vi "Order Ctlrs and Indis.vi"(8 "Error In":errorcluster, 11 "Connector Pane Object Refs":refnum<vi>[][](array[refnum])) -> (0 "Error Out":errorcluster, 2 "Ordered  Indicators":refnum<vi>[](array[refnum]), 3 "Ordered Controls":refnum<vi>[](array[refnum]))   [LabVIEW 2014]
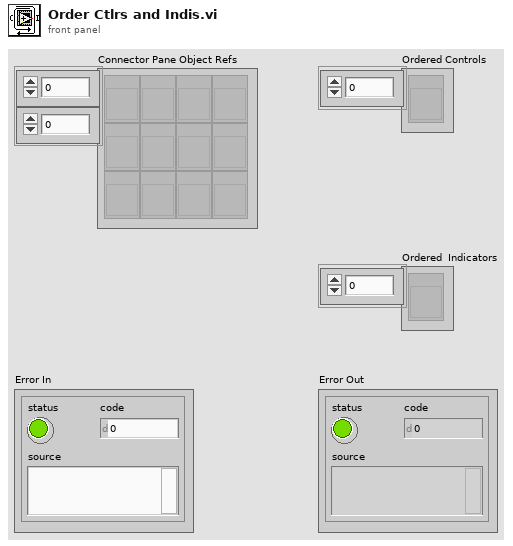
[diagram p1: front panel]
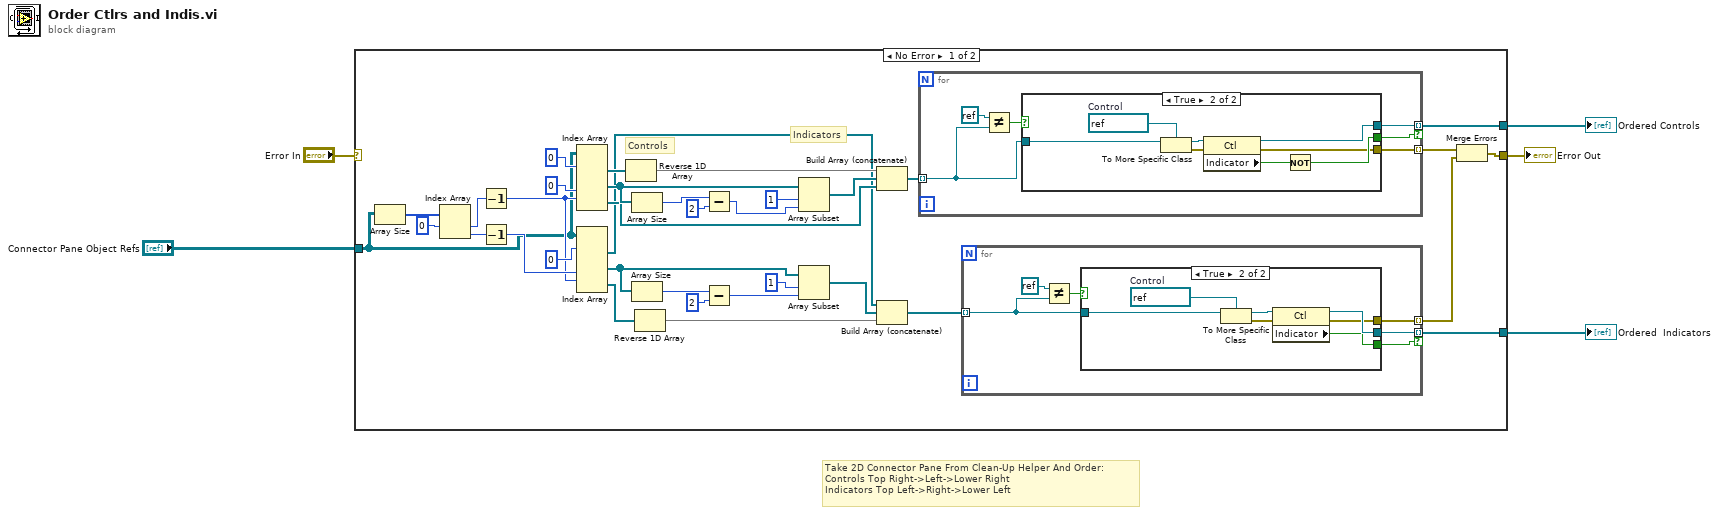
[diagram p0: block diagram]
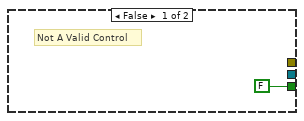
[diagram p2: hidden frame]
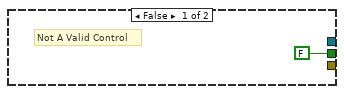
[diagram p3: hidden frame]
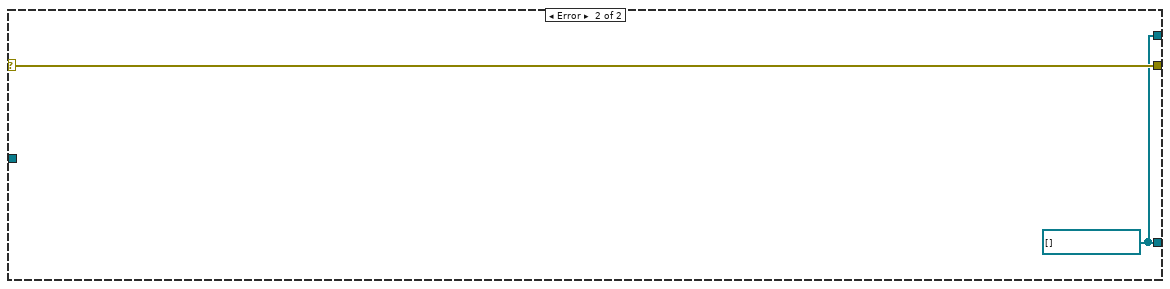
[diagram p4: hidden frame]
diagram:
  # "Take 2D Connector Pane From Clean-Up Helper And Order:\nControls Top Right->Left->Lower Right\nIndicators Top Left->Right->Lower Left"
  n1 = case shown="No Error" "Error In" {
    selector: "Error In" -> [_ w71]
    tunnel: "Connector Pane Object Refs" -> [w13 _]
    tunnel: [w8 w70] -> w4
    tunnel: [w7 w70] -> w3
    tunnel: [w6 w71] -> w1
    frame No Error {
      # "Indicators"
      # "Controls"
      n2 = Array Size(array=w13) -> (size(s)=w32:i32[])
      n3 = Index Array(array=w32, index #1=0 ("index")) -> (element #1=w30:i32, element #2=w25:i32)  [unwired: 1 in]
      n4 = Decrement(x=w30) -> (x-1=w18:i32)
      n5 = Decrement(x=w25) -> (x-1=w24:i32)
      n6 = Index Array(array=w13, index (row) #1=0 ("index (row)"), index (col) #2=0 ("disabled index (col)"), index (row) #3=w18) -> (element #1=w39:refnum<vi>[], element #2=w36:refnum<vi>[], element #3=w27:refnum<vi>[])  [unwired: 3 in]
      n7 = Index Array(array=w13, index (row) #1=0 ("index (row)"), index (col) #2=w24, index (row) #3=w18) -> (element #1=w16:refnum<vi>[], element #2=w19:refnum<vi>[], element #3=w17:refnum<vi>[])  [unwired: 3 in]
      n8 = Reverse 1D Array(array=w39) -> (reversed array=w29:refnum<vi>[])
      n9 = Array Size(array=w36) -> (size(s)=w35:i32)
      n10 = Array Size(array=w19) -> (size(s)=w21:i32)
      n11 = Reverse 1D Array(array=w17) -> (reversed array=w14:refnum<vi>[])
      n12 = Subtract(x=w35, y=2) -> (x-y=w33:i32)
      n13 = Subtract(x=w21, y=2) -> (x-y=w23:i32)
      n14 = Array Subset(array=w36, index=1, length=w33) -> (w28:refnum<vi>[])
      n15 = Array Subset(array=w19, index=1, length=w23) -> (w15:refnum<vi>[])
      n16 = Build Array (concatenate)(w29, w28, w27) -> (w12:refnum<vi>[])
      n17 = Build Array (concatenate)(w16, w15, w14) -> (w11:refnum<vi>[])
      n18 = for {
        tunnel: w12 -> [w56] mode=indexing
        tunnel: [w60] -> w8 mode=indexing if=w59
        tunnel: [w58] -> w10 mode=indexing
        n19 = Not Equal?(x=refnum<k0> refnum, y=w56) -> (x != y?=w55:bool)
        n20 = case shown="True" w55 {
          tunnel: [_ w65] -> w60
          tunnel: [FALSE w64] -> w59
          tunnel: [_ w63] -> w58
          tunnel: w56 -> [_ w62]
          frame False {
            # "Not A Valid Control"
          }
          frame True {
            w69 = refnum<vi> refnum  # Control
            n21 = To More Specific Class(target class=w69, reference=w62) -> (specific class reference=w68:refnum<vi>, error out=w67:errorcluster)  [unwired: 1 in]
            n22 = property class="Ctl"(reference=w68, error in=w67) -> (reference out=w65:refnum<vi>, error out=w63:errorcluster, "Indicator"=w66:bool)
            n23 = Not(x=w66) -> (.not. x?=w64:bool)
          }
        }
      }
      n24 = for {
        tunnel: w11 -> [w41] mode=indexing
        tunnel: [w46] -> w7 mode=indexing if=w45
        tunnel: [w44] -> w9 mode=indexing
        n25 = Not Equal?(x=refnum<k0> refnum, y=w41) -> (x != y?=w42:bool)
        n26 = case shown="True" w42 {
          tunnel: w41 -> [_ w54]
          tunnel: [_ w50] -> w46
          tunnel: [FALSE ("Indicator") w49] -> w45
          tunnel: [_ w48] -> w44
          frame False {
            # "Not A Valid Control"
          }
          frame True {
            w53 = refnum<vi> refnum  # Control
            n27 = To More Specific Class(target class=w53, reference=w54) -> (specific class reference=w52:refnum<vi>, error out=w51:errorcluster)  [unwired: 1 in]
            n28 = property class="Ctl"(reference=w52, error in=w51) -> (reference out=w50:refnum<vi>, error out=w48:errorcluster, "Indicator"=w49:bool)
          }
        }
      }
      n29 = Merge Errors(w10, w9) -> (w6:errorcluster)
    }
    frame Error {
      w70 = refnum<vi>[] []
    }
  }
  "Error Out" <- w1
  "Ordered  Indicators" <- w3
  "Ordered Controls" <- w4
